vi "CD Init_Prepare Inline Data.vi"(8 "error in (no error)":errorcluster, 11 "channels In":T12[](array[typedef]) {"RTs"."Mode Codes"."Words Item Refs" format="%.0x"; "RTs"."Mode Codes"."Timestamp Channel Data Reference" format="%.0x"; "RTs"."subAddresses"."Words Item Refs" format="%.0x"; "RTs"."subAddresses"."Timestamp Channel Data Reference" format="%.0x"; "RTs"."Status Channel Data Reference" format="%.0x"; "RTs"."Command Channels Refs" format="%.0x"; "BC"."Acyclic Frames Trigger Channels Refs" format="%.0x"; "BC"."Command Channels Refs" format="%.0x"; "BC"."messages"."Timestamp Channel Data Reference" format="%.0x"; "BC"."messages"."Status Channel Data Refs" format="%.0x"; "BC"."messages"."Words Item Refs" format="%.0x"; "BC"."messages"."Words Block Data Refs"."Data Reference" format="%.0x"}) -> (0 "error out":errorcluster, 3 "RT Inline Data_Data Description_Channels":T1[](array[typedef]) {"Broadcast Frame Descriptors"."RTs"."Status Channel Ref" format="%.0x"; "Broadcast Frame Descriptors"."RTs"."Timestamp Channel Data Reference" format="%.0x"; "Broadcast Frame Descriptors"."BC"."Status Channel Refs" format="%.0x"; "Broadcast Frame Descriptors"."BC"."Words Block Data Refs"."Data Reference" format="%.0x"; "Broadcast Frame Descriptors"."BC"."Timestamp Channel Data Reference" format="%.0x"; "Frame Drescriptors"."RT"."Status Channel Ref" format="%.0x"; "Frame Drescriptors"."RT"."Words Block Data Refs"."Data Reference" format="%.0x"; "Frame Drescriptors"."RT"."Timestamp Channel Data Reference" format="%.0x"; "Frame Drescriptors"."BC"."Status Channel Refs" format="%.0x"; "Frame Drescriptors"."BC"."Words Block Data Refs"."Data Reference" format="%.0x"; "Frame Drescriptors"."BC"."Timestamp Channel Data Reference" format="%.0x"})   [LabVIEW 2017, in "Ballard MIL-1553 Engine.lvlib"]
uses:
  Ballard MIL-1553 Engine.lvlib
  Shared/Controls and Global/RT Channel.ctl
  Shared/Controls and Global/RT BC.ctl
  <vilib>/NI Veristand/Custom Device API/Custom Device Item Ref.ctl
  Shared/Controls and Global/RT Message.ctl
  Shared/Controls and Global/RT messageType.ctl
  Shared/Controls and Global/RT CWD1.ctl
  Shared/Controls and Global/RT CWD2.ctl
  <vilib>/NI Veristand/Custom Device API/Data Reference.ctl
  <vilib>/NI Veristand/Custom Device API/Block Data Reference.ctl
  Shared/Controls and Global/RT Remote Terminal.ctl
  Shared/Controls and Global/RT Remote Terminal_rtMode.ctl
  Shared/Controls and Global/RT Remote Terminal_RT subAddress.ctl
  Shared/Controls and Global/RT Remote Terminal_RT direction.ctl
  Shared/Controls and Global/RT Remote Terminal_RT Mode Code.ctl
  Controls/RT Inline Data_Data Description_Channel.ctl
  Controls/RT Inline Frame Descriptor.ctl
  Controls/RT Inline Frame Descriptor_BC.ctl
  Controls/RT Inline Frame Descriptor_RT.ctl
  Controls/RT Inline Broadcast Frame Descriptor.ctl
  <vilib>/NI VeriStand/Custom Device API/Custom Device API.lvlib
  Shared/Ballard 1553 Shared.lvlib
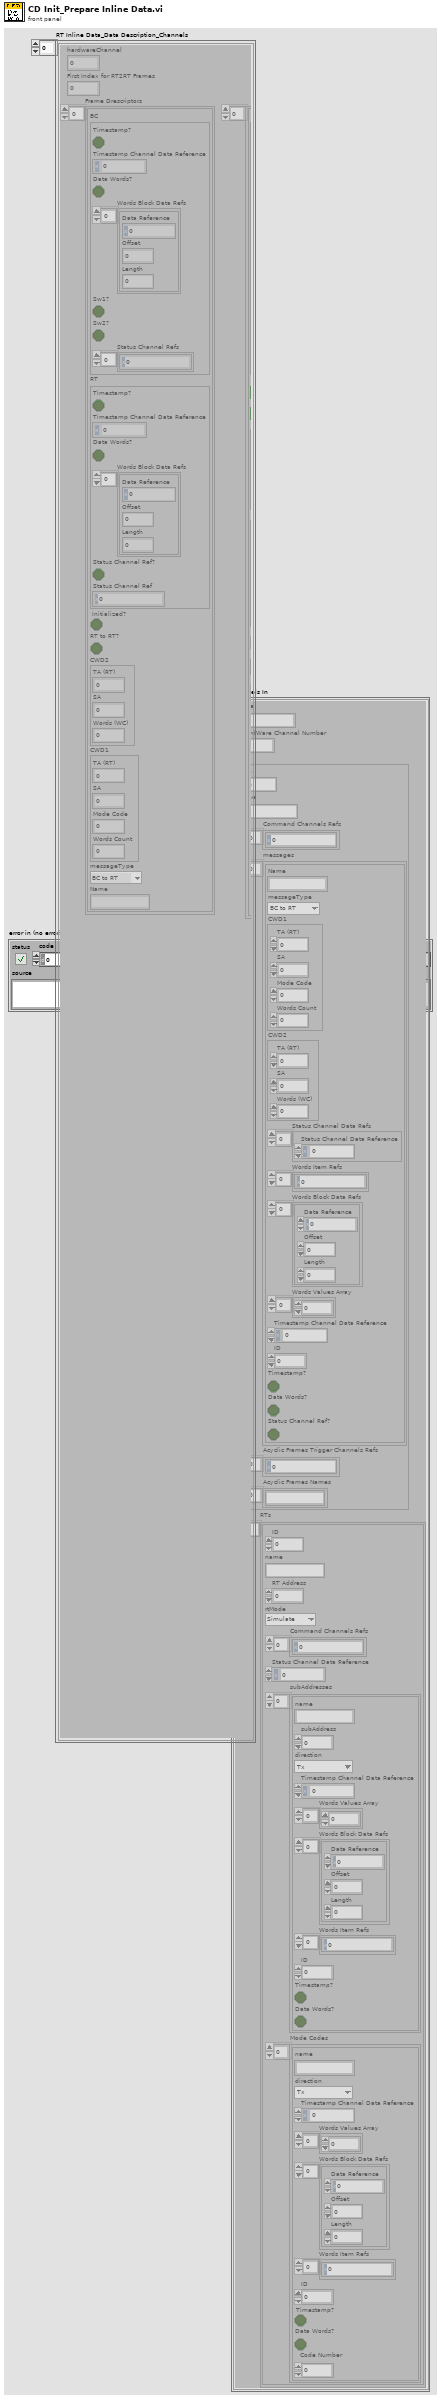
[diagram p1: front panel]
types:
  T1 = typedef "Ballard MIL-1553 Engine.lvlib/RT Inline Data_Data Description_Channel.ctl" = cluster{"hardwareChannel":u16, "First Index for RT2RT Frames":i32, "Frame Drescriptors":T2[], "Broadcast Frame Descriptors":T11[]}
  T2 = typedef "Ballard MIL-1553 Engine.lvlib/RT Inline Frame Descriptor.ctl" = cluster{"BC":T3, "RT":T7, "Initialized?":bool, "RT to RT?":bool, "CWD2":T8, "CWD1":T9, "messageType":T10, "Name":string}
  T3 = typedef "Ballard MIL-1553 Engine.lvlib/RT Inline Frame Descriptor_BC.ctl" = cluster{"Timestamp?":bool, "Timestamp Channel Data Reference":T4, "Data Words?":bool, "Words Block Data Refs":T5[], "Sw1?":bool, "Sw2?":bool, "Status Channel Refs":T6[]}
  T4 = typedef "Custom Device API.lvlib/Data Reference.ctl" = i32
  T5 = typedef "Custom Device API.lvlib/Block Data Reference.ctl" = cluster{"Data Reference":T4, "Offset":u64, "Length":u64}
  T6 = typedef "Custom Device API.lvlib/Custom Device Item Ref.ctl" = u64
  T7 = typedef "Ballard MIL-1553 Engine.lvlib/RT Inline Frame Descriptor_RT.ctl" = cluster{"Timestamp?":bool, "Timestamp Channel Data Reference":T4, "Data Words?":bool, "Words Block Data Refs":T5[], "Status Channel Ref?":bool, "Status Channel Ref":T6}
  T8 = typedef "Ballard 1553 Shared.lvlib/RT CWD2.ctl" = cluster{"TA (RT)":i8, "SA":i8, "Words (WC)":i8}
  T9 = typedef "Ballard 1553 Shared.lvlib/RT CWD1.ctl" = cluster{"TA (RT)":i8, "SA":i8, "Mode Code":i8, "Words Count":i8}
  T10 = typedef "Ballard 1553 Shared.lvlib/RT messageType.ctl" = enum16{"BC to RT", "RT to BC", "RT to RT", "MC (Rx)", "MC (Tx)"}
  T11 = typedef "Ballard MIL-1553 Engine.lvlib/RT Inline Broadcast Frame Descriptor.ctl" = cluster{"BC":T3, "Initialized?":bool, "RT to RT?":bool, "CWD2":T8, "CWD1":T9, "messageType":T10, "Name":string, "RTs":T7[]}
  T12 = typedef "Ballard 1553 Shared.lvlib/RT Channel.ctl" = cluster{"name":string, "hardWare Channel Number":u16, "BC":T13, "RTs":T15[]}
  T13 = typedef "Ballard 1553 Shared.lvlib/RT BC.ctl" = cluster{"ID":i32, "name":string, "Command Channels Refs":T6[], "messages":T14[], "Acyclic Frames Trigger Channels Refs":T6[], "Acyclic Frames Names":string[]}
  T14 = typedef "Ballard 1553 Shared.lvlib/RT Message.ctl" = cluster{"Name":string, "messageType":T10, "CWD1":T9, "CWD2":T8, "Status Channel Data Refs":T4[], "Words Item Refs":T6[], "Words Block Data Refs":T5[], "Words Values Array":u16[], "Timestamp Channel Data Reference":T4, "ID":i32, "Timestamp?":bool, "Data Words?":bool, "Status Channel Ref?":bool}
  T15 = typedef "Ballard 1553 Shared.lvlib/RT Remote Terminal.ctl" = cluster{"ID":i32, "name":string, "RT Address":i32, "rtMode":T16, "Command Channels Refs":T6[], "Status Channel Data Reference":T4, "subAddresses":T17[], "Mode Codes":T19[]}
  T16 = typedef "Ballard 1553 Shared.lvlib/RT Remote Terminal_rtMode.ctl" = enum16{"Simulate", "Monitor", "Disable"}
  T17 = typedef "Ballard 1553 Shared.lvlib/RT Remote Terminal_RT subAddress.ctl" = cluster{"name":string, "subAddress":i8, "direction":T18, "Timestamp Channel Data Reference":T4, "Words Values Array":u16[], "Words Block Data Refs":T5[], "Words Item Refs":T6[], "ID":i32, "Timestamp?":bool, "Data Words?":bool}
  T18 = typedef "Ballard 1553 Shared.lvlib/RT Remote Terminal_RT direction.ctl" = enum16{"Tx", "Rx"}
  T19 = typedef "Ballard 1553 Shared.lvlib/RT Remote Terminal_RT Mode Code.ctl" = cluster{"name":string, "direction":T18, "Timestamp Channel Data Reference":T4, "Words Values Array":u16[], "Words Block Data Refs":T5[], "Words Item Refs":T6[], "ID":i32, "Timestamp?":bool, "Data Words?":bool, "Code Number":i32}
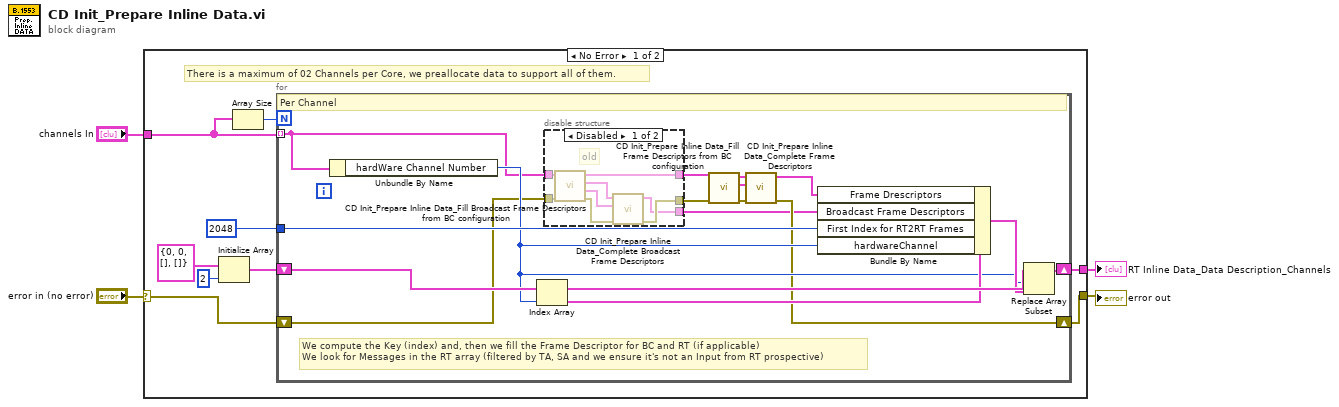
[diagram p0: block diagram]
diagram:
  n1 = case shown="No Error" "error in (no error)" {
    selector: "error in (no error)" -> [w6 w40]
    tunnel: [w5 w40] -> w3
    tunnel: "channels In" -> [w12 _]
    tunnel: [w8 _] -> w1
    frame No Error {
      # "There is a maximum of 02 Channels per Core, we preallocate data to support all of them."
      n2 = Initialize Array(T1 {"hardwareChannel"=0, "First Index for RT2RT Frames"=0, "Frame Drescriptors"=[], "Broadcast Frame Descriptors"=[]} ("RT Inline Data_Data Description_Channel"), 2 ("dimension size")) -> (w9:T1[])
      n3 = Array Size(array=w12) -> (size(s)=w13:i32)
      n4 = for {
        N: w13 -> [_]
        tunnel: w12 -> [w18] mode=indexing
        shift-right: [w28] -> w8
        shift-left: w9 -> [w29]
        tunnel: 2048 ("dimension size") -> [w25]
        shift-right: [w21] -> w5
        shift-left: w6 -> [w17]
        # "We compute the Key (index) and, then we fill the Frame Descriptor for BC and RT (if applicable)\nWe look for Messages in the RT array (filtered by TA, SA and we ensure it's not an Input from RT prospective)"
        # "Per Channel"
        n5 = Unbundle By Name(w18) -> ("hardWare Channel Number"=w24:u16)
        n6 = Index Array(array=w29, index=w24) -> (element=w26:T1)
        n7 = disable-structure shown="Disabled" {
          disable-tunnel: w18 -> [w37 w39]
          disable-tunnel: w17 -> [w36 w38]
          disable-tunnel: [w35 w39] -> w16
          disable-tunnel: [w33 w38] -> w15
          disable-tunnel: [w32 _] -> w14
          frame Disabled {
            # "old"
            n8 = call "CD Init_Prepare Inline Data_Fill Broadcast Frame Descriptors from BC configuration.vi"("error in (no error)"=w36, "RT Channel In"=w37) -> ("error out"=w34:errorcluster, "Broadcast Frame Descriptors Out"=w30:T11[], "RTs Out"=w31:T15[], "RT Channel Out"=w35:T12)  [unwired: 6 in]
            n9 = call "CD Init_Prepare Inline Data_Complete Broadcast Frame Descriptors.vi"("error in (no error)"=w34, "Broadcast Frame Descriptors In"=w30, "RTs In"=w31) -> ("error out"=w33:errorcluster, "Broadcast Frame Descriptors Out"=w32:T11[])  [unwired: 7 in]
          }
          frame Enabled {
            # "New"
          }
        }
        n10 = call "CD Init_Prepare Inline Data_Fill Frame Descriptors from BC configuration.vi"("error in (no error)"=w15, "RT Channel In"=w16) -> ("error out"=w20:errorcluster, "RTs"=w23:T15[], "Frames Descriptors Out"=w22:T2[])  [unwired: 7 in]
        n11 = call "CD Init_Prepare Inline Data_Complete Frame Descriptors.vi"("error in (no error)"=w20, "RTs In"=w23, "Frames Descriptors In"=w22) -> ("error out"=w21:errorcluster, "Frames Descriptors Out"=w19:T2[])  [unwired: 7 in]
        n12 = Bundle By Name(cluster=w26, "Frame Drescriptors"=w19, "Broadcast Frame Descriptors"=w14, "First Index for RT2RT Frames"=w25, "hardwareChannel"=w24) -> (w27:T1)
        n13 = Replace Array Subset(array=w29, new element=w27, index=w24) -> (w28:T1[])
      }
    }
    frame Error {
    }
  }
  "error out" <- w3
  "RT Inline Data_Data Description_Channels" <- w1
